vi "ROIConfig.vi"(8 "ROI In":T1 {"Contours"."Type" items=["No Selection", "Point", "Line", "Rectangle", "Oval", "Polygon", "Freehand Region", "Annulus", "Unused2", "Unused3", "Broken Line", "Freehand Line", "Rotated Rectangle"]}, 10 "Clamped Image":T2, 11 "Improved threshold":T2) -> (0 "ROI  Out":T1 {"Contours"."Type" items=["No Selection", "Point", "Line", "Rectangle", "Oval", "Polygon", "Freehand Region", "Annulus", "Unused2", "Unused3", "Broken Line", "Freehand Line", "Rotated Rectangle"]}, 3 "Orientation":dbl)   [LabVIEW 2015]
uses:
  <vilib>/vision/Image Controls.llb/IMAQ Image.ctl
  <vilib>/vision/NI_Vision_Development_Module.lvlib
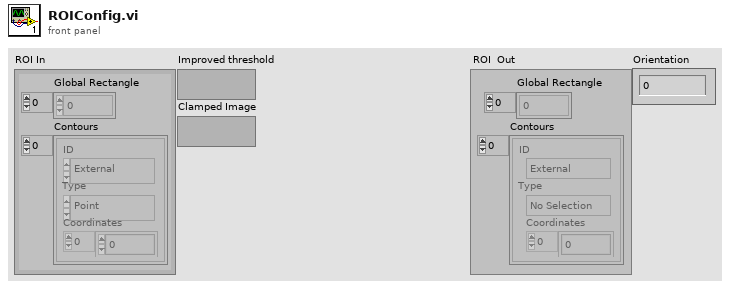
[diagram p1: front panel]
types:
  T1 = typedef "ROI Descriptor" = cluster{"Global Rectangle":i32[], "Contours":cluster{"ID":enum32{"External", "Internal"}, "Type":u32, "Coordinates":i32[]}[]}
  T2 = typedef "IMAQ Image.ctl" = refnum<image>
  T3 = cluster{"Area":dbl, "Number of Holes":dbl, "Bounding Rect":cluster{"Left":dbl, "Top":dbl, "Right":dbl, "Bottom":dbl}, "Center of Mass":cluster{"X":dbl, "Y":dbl}, "Orientation":dbl, "Dimensions":cluster{"Width":dbl, "Height":dbl}}[]
  T4 = cluster{"Area":dbl, "Number of Holes":dbl, "Bounding Rect":cluster{"Left":dbl, "Top":dbl, "Right":dbl, "Bottom":dbl}, "Center of Mass":cluster{"X":dbl, "Y":dbl}, "Orientation":dbl, "Dimensions":cluster{"Width":dbl, "Height":dbl}}
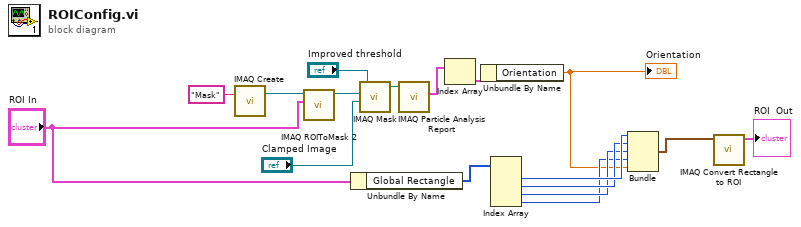
[diagram p0: block diagram]
diagram:
  n1 = call "IMAQ Create"("Image Name"="Mask") -> ("New Image"=w10:T2)  [unwired: 4 in, 1 out]
  n2 = call "IMAQ ROIToMask 2"("ROI Descriptor"="ROI In", "Image"=w10) -> ("Image Out"=w9:T2)  [unwired: 7 in, 2 out]
  n3 = Unbundle By Name("ROI In") -> ("Global Rectangle"=w16:i32[])
  n4 = call "IMAQ Mask"("Image Dst"="Clamped Image", "Image Mask"=w9, "Image Src"="Improved threshold") -> ("Image Dst Out"=w7:T2)  [unwired: 2 in, 1 out]
  n5 = call "IMAQ Particle Analysis Report"("Image"=w7) -> ("Particle Reports (Pixels)"=w17:T3)  [unwired: 5 in, 5 out]
  n6 = Index Array(array=w17) -> (element=w2:T4)  [unwired: 1 in]
  n7 = Unbundle By Name(w2) -> ("Orientation"=w1:dbl)
  "Orientation" <- w1
  n8 = Index Array(array=w16) -> (element #1=w14:i32, element #2=w13:i32, element #3=w12:i32, element #4=w4:i32)  [unwired: 4 in]
  n9 = Bundle(w14, w13, w12, w4, "Orientation"=w1) -> (w15:cluster{i32, i32, i32, i32, "Orientation":dbl})  [unwired: 1 in]
  n10 = call "IMAQ Convert Rectangle to ROI"("Rectangle"=w15) -> ("ROI Descriptor"=→"ROI  Out":T1)  [unwired: 8 in, 1 out]
